vi "Report Error.vi"(8 "error in (no error)":errorcluster) -> ()   [LabVIEW 2014]
uses:
  Globals.vi
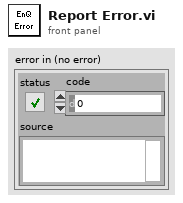
[diagram p1: front panel]
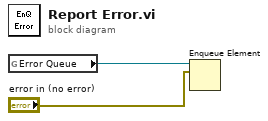
[diagram p0: block diagram]
diagram:
  n1 = global read "Globals.vi" "Error Queue"() -> (w2:refnum<queue>)
  n2 = Enqueue Element(queue=w2, element="error in (no error)") -> ()  [unwired: 2 in, 3 out]
